vi "Modify Data format to R2.vi"(6 "Current set number in one current mode":i32=48, 7 "Scan number":i32=10, 8 "modified error":errorcluster, 9 "modified Data path":path, 10 "original error":errorcluster, 11 "original Data path":path) -> ()   [LabVIEW 2023]
uses:
  <vilib>/Utility/error.llb/DialogType.ctl
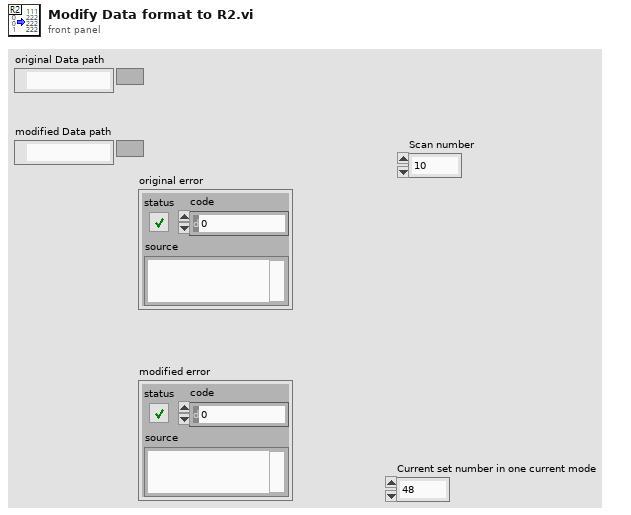
[diagram p1: front panel]
types:
  T1 = enum16{"open", "replace", "create", "open or create", "replace or create", "replace or create with confirmation"}
  T2 = typedef "DialogType.ctl" = u16
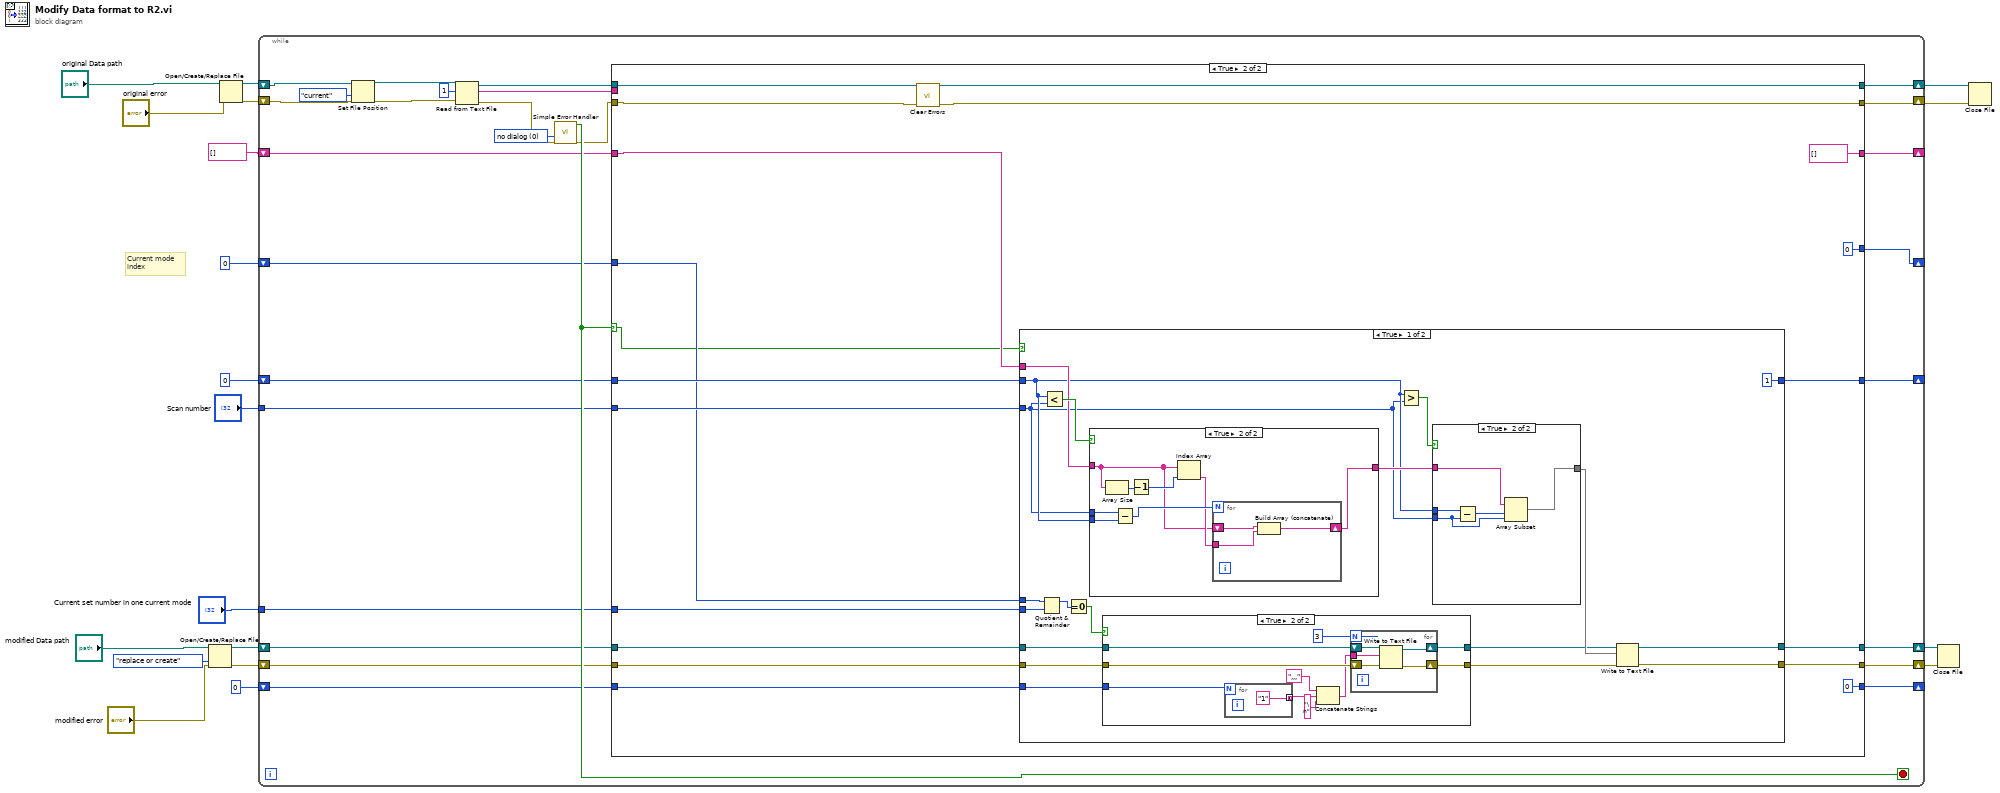
[diagram p0: block diagram]
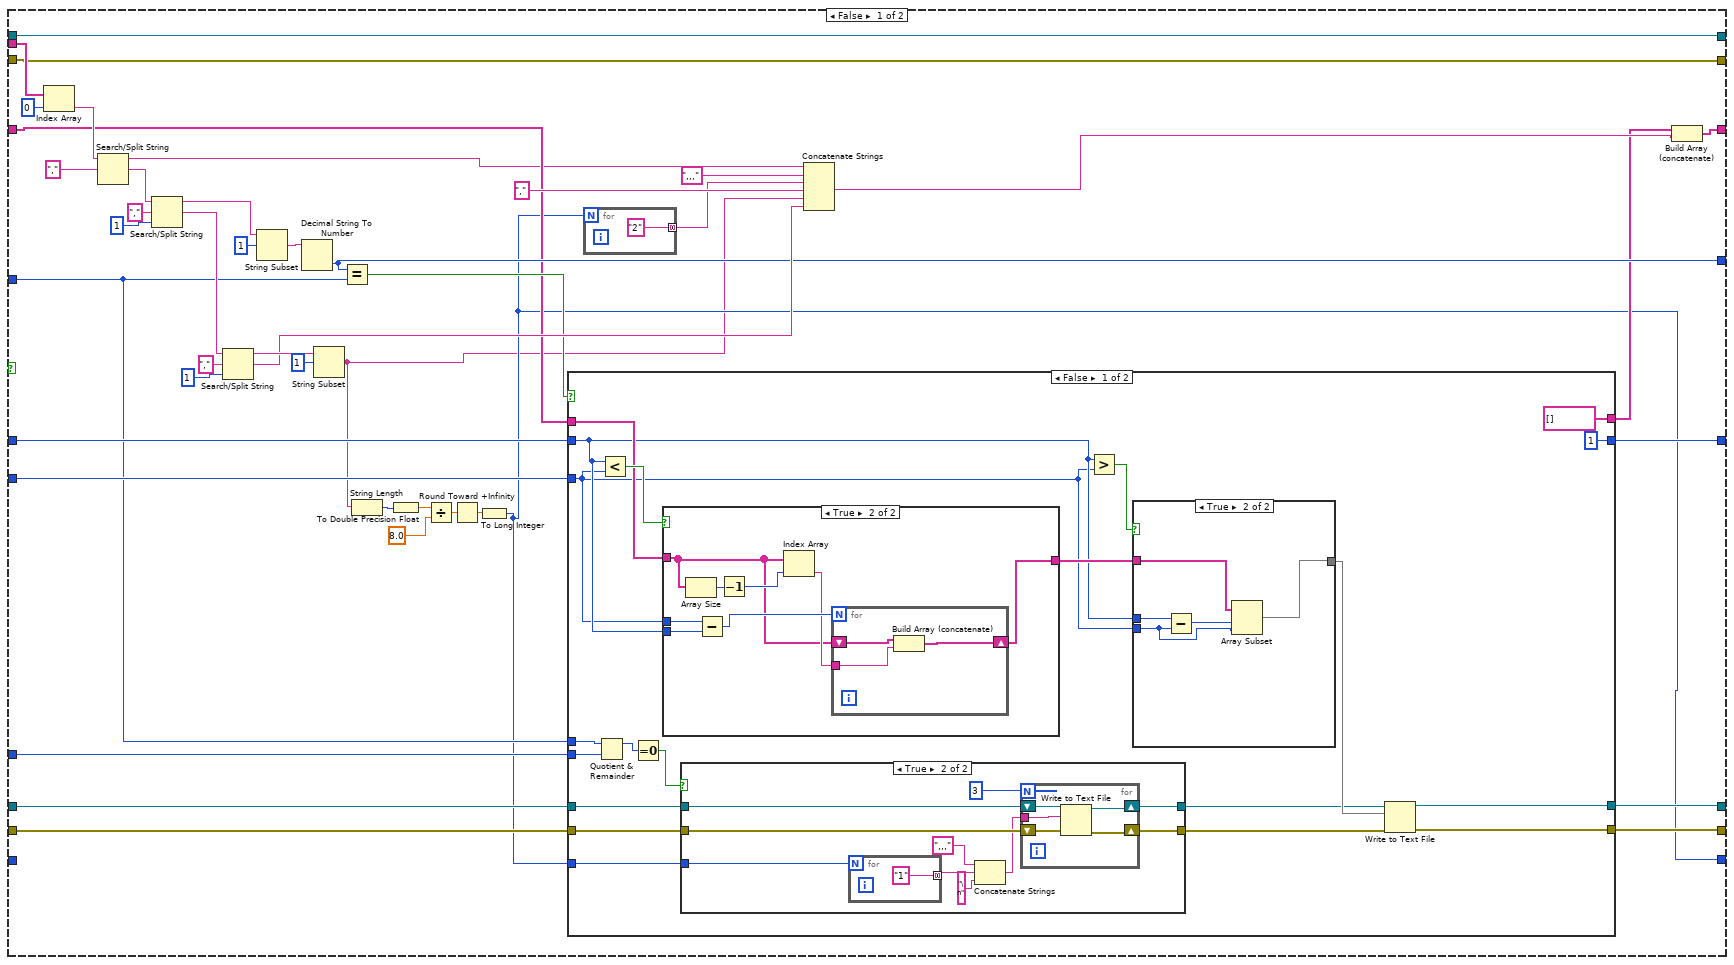
[diagram p2: hidden frame]
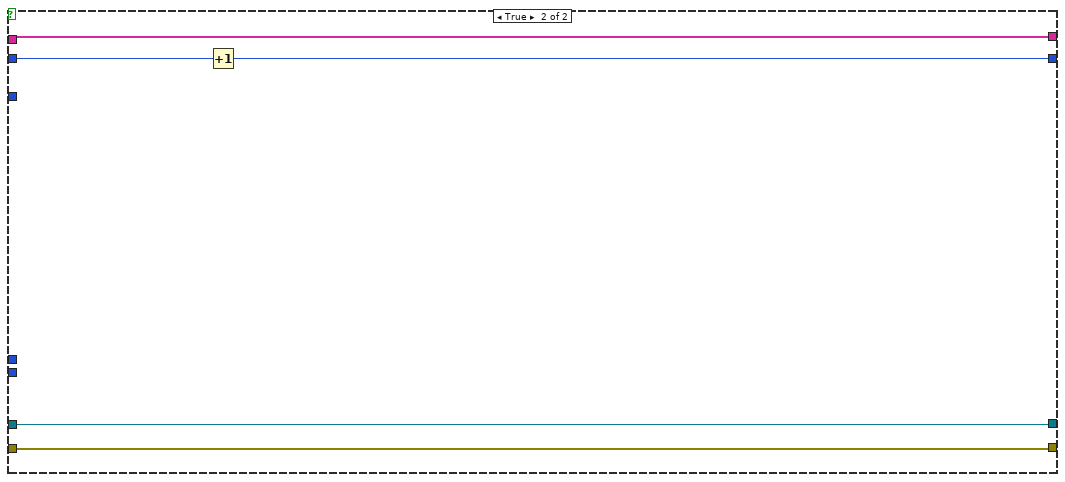
[diagram p6: hidden frame]
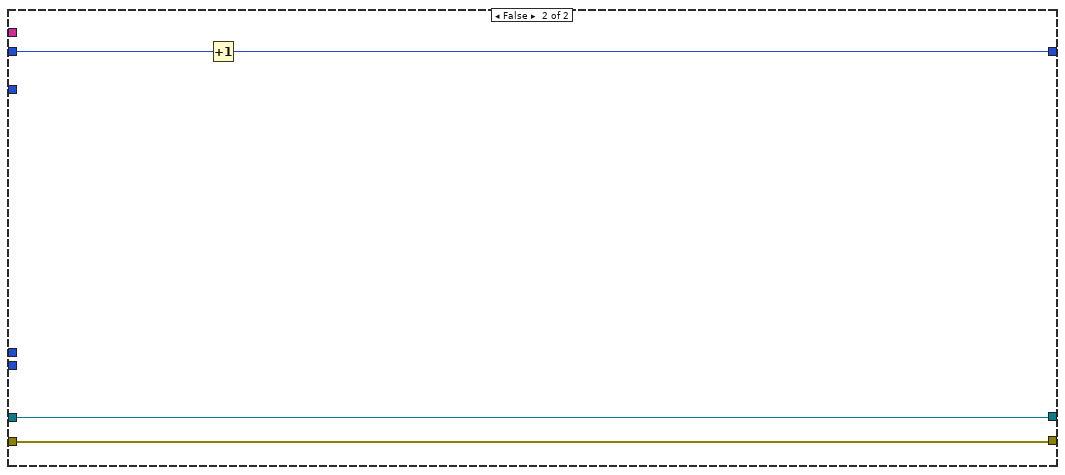
[diagram p10: hidden frame]
diagram:
  # "Current mode\nindex"
  n1 = Open/Create/Replace File(file path (use dialog)="modified Data path", error in="modified error", operation (0:open)=T1."replace or create") -> (refnum out=w16:refnum<file>, error out=w15:errorcluster)  [unwired: 3 in, 1 out]
  n2 = Open/Create/Replace File(file path (use dialog)="original Data path", error in="original error") -> (refnum out=w17:refnum<file>, error out=w18:errorcluster)  [unwired: 4 in, 1 out]
  n3 = while {
    shift-right: [w39] -> w9
    shift-left: w18 -> [w46]
    shift-right: [w38] -> w19
    shift-left: w17 -> [w37]
    shift-right: [w32] -> w11
    shift-left: w16 -> [w34]
    shift-right: [w31] -> w10
    shift-left: w15 -> [w33]
    shift-right: [w20] -> _
    shift-left: string[] [] ("element") -> [w29]
    shift-right: [w25] -> _
    shift-left: 0 ("number") -> [w28]
    shift-right: [w26] -> _
    shift-left: 0 ("number") -> [w27]
    tunnel: "Scan number" -> [w24]
    tunnel: "Current set number in one current mode" -> [w23]
    shift-right: [w22] -> _
    shift-left: 0 ("32bit integer") -> [w21]
    stop <- w43 stop-if-true
    w44 = T2 0 items=["no dialog", "OK message", "continue or stop message", "OK message + warnings", "continue/stop + warnings"] ("type of dialog (OK msg:1)")
    n4 = Set File Position(refnum=w37, from (0:start)=enum16{"start", "end", "current"}."current", error in=w46) -> (refnum out=w36:refnum<file>, error out=w35:errorcluster)  [unwired: 1 in]
    n5 = Read from Text File(file (use dialog)=w36, count=1, error in=w35) -> (refnum out=w41:refnum<file>, text=w42:string[], error out=w40:errorcluster)  [unwired: 1 in, 1 out]
    n6 = call <vilib>:"Simple Error Handler.vi"("type of dialog (OK msg:1)"=w44, "error in (no error)"=w40) -> ("error?"=w43:bool, "error out"=w30:errorcluster)  [unwired: 3 in, 3 out]
    n7 = case shown="True" w43 {
      selector: w43 -> [_ w158]
      tunnel: w42 -> [w86 _]
      tunnel: w41 -> [w84 w171]
      tunnel: w30 -> [w83 w160]
      tunnel: [w84 w171] -> w38
      tunnel: [w83 w159] -> w39
      tunnel: w34 -> [w64 w166]
      tunnel: w33 -> [w63 w165]
      tunnel: [w62 w164] -> w32
      tunnel: [w61 w163] -> w31
      tunnel: w29 -> [w66 w167]
      tunnel: w28 -> [w60 w162]
      tunnel: w27 -> [w71 w170]
      tunnel: [w70 w169] -> w26
      tunnel: [w69 0] -> w25
      tunnel: w24 -> [w67 w168]
      tunnel: w23 -> [w59 w161]
      tunnel: [w50 0] -> w22
      tunnel: w21 -> [_ w155]
      tunnel: [w49 string[] [] ("element")] -> w20
      frame False {
        n8 = Index Array(array=w86, index=0) -> (element=w82:string)
        n9 = Search/Split String(string=w82, search string/char (-)=",") -> (substring before match=w53:string, match + rest of string=w91:string)  [unwired: 1 in, 1 out]
        n10 = Search/Split String(string=w91, search string/char (-)=",", offset (0)=1) -> (substring before match=w74:string, match + rest of string=w79:string)  [unwired: 1 out]
        n11 = Search/Split String(string=w79, search string/char (-)=",", offset (0)=1) -> (substring before match=w78:string, match + rest of string=w76:string)  [unwired: 1 out]
        n12 = String Subset(string=w74, offset (0)=1) -> (substring=w73:string)  [unwired: 1 in]
        n13 = Decimal String To Number(string=w73) -> (number=w69:i32)  [unwired: 2 in, 1 out]
        n14 = String Subset(string=w78, offset (0)=1) -> (substring=w48:string)  [unwired: 1 in]
        n15 = Equal?(x=w69, y=w60) -> (x = y?=w72:bool)
        n16 = String Length(string=w48) -> (length=w56:i32)
        n17 = To Double Precision Float(number=w56) -> (double precision float=w57:dbl)
        n18 = Divide(x=w57, y=8.0) -> (x/y=w58:dbl)
        n19 = Round Toward +Infinity(x=w58) -> (ceil(x): smallest int >= x=w54:dbl)
        n20 = To Long Integer(number=w54) -> (32bit integer=w50:i32)
        n21 = case shown="False" w72 {
          tunnel: [1 w152] -> w70
          tunnel: w71 -> [w106 w153]
          tunnel: w67 -> [w105 _]
          tunnel: w66 -> [w109 w151]
          tunnel: [string[] [] ("element") w151] -> w65
          tunnel: w64 -> [w97 w150]
          tunnel: w63 -> [w96 w149]
          tunnel: [w103 w150] -> w62
          tunnel: [w102 w149] -> w61
          tunnel: w60 -> [w101 _]
          tunnel: w59 -> [w100 _]
          tunnel: w50 -> [w93 _]
          frame False {
            n22 = Quotient & Remainder(x=w101, y=w100) -> (x-y*floor(x/y)=w99:i32)  [unwired: 1 out]
            n23 = Less?(x=w106, y=w105) -> (x < y?=w110:bool)
            n24 = Equal To 0?(x=w99) -> (x = 0?=w98:bool)
            n25 = case shown="True" w110 {
              tunnel: w109 -> [w137 w139]
              tunnel: w105 -> [_ w143]
              tunnel: w106 -> [_ w142]
              tunnel: [w137 w138] -> w107
              frame False {
              }
              frame True {
                n26 = Array Size(array=w139) -> (size(s)=w145:i32)
                n27 = Subtract(x=w143, y=w142) -> (x-y=w141:i32)
                n28 = Decrement(x=w145) -> (x-1=w144:i32)
                n29 = Index Array(array=w139, index=w144) -> (element=w140:string)
                n30 = for {
                  N: w141 -> [_]
                  tunnel: w140 -> [w146]
                  shift-right: [w147] -> w138
                  shift-left: w139 -> [w148]
                  n31 = Build Array (concatenate)(w148, w146) -> (w147:string[])
                }
              }
            }
            n32 = case shown="True" w98 {
              tunnel: w97 -> [w114 w120]
              tunnel: w96 -> [w113 w119]
              tunnel: [w114 w117] -> w95
              tunnel: [w113 w116] -> w94
              tunnel: w93 -> [_ w115]
              frame False {
              }
              frame True {
                n33 = for {
                  N: w115 -> [_]
                  tunnel: ["1" ("search string/char (-)")] -> w123 mode=concatenating
                }
                n34 = Concatenate Strings(",,," ("string"), w123, "\n" ("string")) -> (w118:string)
                n35 = for {
                  N: 3 -> [_]
                  shift-right: [w127] -> w117
                  shift-left: w120 -> [w130]
                  tunnel: w118 -> [w128]
                  shift-right: [w126] -> w116
                  shift-left: w119 -> [w129]
                  n36 = Write to Text File(file (use dialog)=w130, text=w128, error in=w129) -> (refnum out=w127:refnum<file>, error out=w126:errorcluster)  [unwired: 1 in, 1 out]
                }
              }
            }
            n37 = Greater?(x=w106, y=w105) -> (0:w108:bool)
            n38 = case shown="True" w108 {
              tunnel: w107 -> [w131 w135]
              tunnel: w106 -> [_ w136]
              tunnel: w105 -> [_ w133]
              tunnel: [w131 w132] -> w104
              frame False {
              }
              frame True {
                n39 = Subtract(x=w136, y=w133) -> (x-y=w134:i32)
                n40 = Array Subset(array=w135, index=w134, length=w133) -> (w132:string[])
              }
            }
            n41 = Write to Text File(file (use dialog)=w95, text=w104, error in=w94) -> (refnum out=w103:refnum<file>, error out=w102:errorcluster)  [unwired: 1 in, 1 out]
          }
          frame True {
            n42 = Increment(x=w153) -> (x+1=w152:i32)
          }
        }
        n43 = for {
          N: w50 -> [_]
          tunnel: ["2" ("search string/char (-)")] -> w51 mode=concatenating
        }
        n44 = Concatenate Strings(w53, ",,," ("string"), w51, "," ("string"), w48, w76) -> (w68:string)
        n45 = Build Array (concatenate)(w65, w68) -> (w49:string[])
      }
      frame True {
        n46 = call <vilib>:"Clear Errors.vi"("error in (no error)"=w160) -> ("error out"=w159:errorcluster)  [unwired: 5 in, 1 out]
        n47 = case shown="True" w158 {
          tunnel: [1 w229] -> w169
          tunnel: w170 -> [w185 w230]
          tunnel: w168 -> [w184 _]
          tunnel: w167 -> [w188 _]
          tunnel: w166 -> [w176 w228]
          tunnel: w165 -> [w175 w227]
          tunnel: [w182 w228] -> w164
          tunnel: [w181 w227] -> w163
          tunnel: w162 -> [w180 _]
          tunnel: w161 -> [w179 _]
          tunnel: w155 -> [w172 _]
          frame True {
            n48 = Quotient & Remainder(x=w180, y=w179) -> (x-y*floor(x/y)=w178:i32)  [unwired: 1 out]
            n49 = Less?(x=w185, y=w184) -> (x < y?=w189:bool)
            n50 = Equal To 0?(x=w178) -> (x = 0?=w177:bool)
            n51 = case shown="True" w189 {
              tunnel: w188 -> [w215 w217]
              tunnel: w184 -> [_ w221]
              tunnel: w185 -> [_ w220]
              tunnel: [w215 w216] -> w186
              frame False {
              }
              frame True {
                n52 = Array Size(array=w217) -> (size(s)=w223:i32)
                n53 = Subtract(x=w221, y=w220) -> (x-y=w219:i32)
                n54 = Decrement(x=w223) -> (x-1=w222:i32)
                n55 = Index Array(array=w217, index=w222) -> (element=w218:string)
                n56 = for {
                  N: w219 -> [_]
                  tunnel: w218 -> [w224]
                  shift-right: [w225] -> w216
                  shift-left: w217 -> [w226]
                  n57 = Build Array (concatenate)(w226, w224) -> (w225:string[])
                }
              }
            }
            n58 = case shown="True" w177 {
              tunnel: w176 -> [w192 w198]
              tunnel: w175 -> [w191 w197]
              tunnel: [w192 w195] -> w174
              tunnel: [w191 w194] -> w173
              tunnel: w172 -> [_ w193]
              frame False {
              }
              frame True {
                n59 = for {
                  N: w193 -> [_]
                  tunnel: ["1" ("search string/char (-)")] -> w201 mode=concatenating
                }
                n60 = Concatenate Strings(",,," ("string"), w201, "\n" ("string")) -> (w196:string)
                n61 = for {
                  N: 3 -> [_]
                  shift-right: [w205] -> w195
                  shift-left: w198 -> [w208]
                  tunnel: w196 -> [w206]
                  shift-right: [w204] -> w194
                  shift-left: w197 -> [w207]
                  n62 = Write to Text File(file (use dialog)=w208, text=w206, error in=w207) -> (refnum out=w205:refnum<file>, error out=w204:errorcluster)  [unwired: 1 in, 1 out]
                }
              }
            }
            n63 = Greater?(x=w185, y=w184) -> (0:w187:bool)
            n64 = case shown="True" w187 {
              tunnel: w186 -> [w209 w213]
              tunnel: w185 -> [_ w214]
              tunnel: w184 -> [_ w211]
              tunnel: [w209 w210] -> w183
              frame False {
              }
              frame True {
                n65 = Subtract(x=w214, y=w211) -> (x-y=w212:i32)
                n66 = Array Subset(array=w213, index=w212, length=w211) -> (w210:string[])
              }
            }
            n67 = Write to Text File(file (use dialog)=w174, text=w183, error in=w173) -> (refnum out=w182:refnum<file>, error out=w181:errorcluster)  [unwired: 1 in, 1 out]
          }
          frame False {
            n68 = Increment(x=w230) -> (x+1=w229:i32)
          }
        }
      }
    }
  }
  n69 = Close File(refnum=w11, error in=w10) -> ()  [unwired: 2 out]
  n70 = Close File(refnum=w19, error in=w9) -> ()  [unwired: 2 out]
